vi "Append Usage.vi"(9 "Class":string, 10 "VIs":refnum<vi>[](array[refnum]), 11 "Class Relations Map":T1(c390)) -> (3 "Class Relations Map Out":T1(c390))   [LabVIEW 2019]
uses:
  <vilib>/Utility/traverseref.llb/TRef TravTarget.ctl
  <vilib>/Utility/miscctls.llb/LVMapReplaceAction.ctl
  <vilib>/Utility/traverseref.llb/VI Scripting - Traverse.lvlib
  <vilib>/Utility/Data Type/NI_Data Type.lvlib
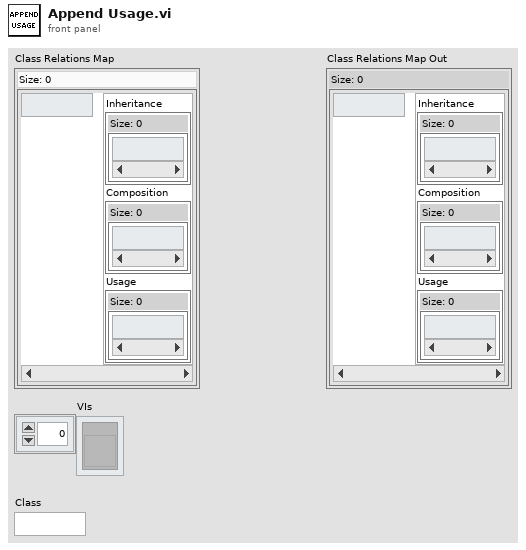
[diagram p1: front panel]
types:
  T1 = map{string, cluster{"Inheritance":set{string}, "Composition":set{string}, "Usage":set{string}}}
  T2 = typedef "TRef TravTarget.ctl" = enum16{"FP", "BD", "Other"}
  T3 = typedef "LVMapReplaceAction.ctl" = enum32{"Modify Entry only if found", "Add or Modify Entry", "Delete Entry"}
  T4 = cluster{"Inheritance":set{string}, "Composition":set{string}, "Usage":set{string}}
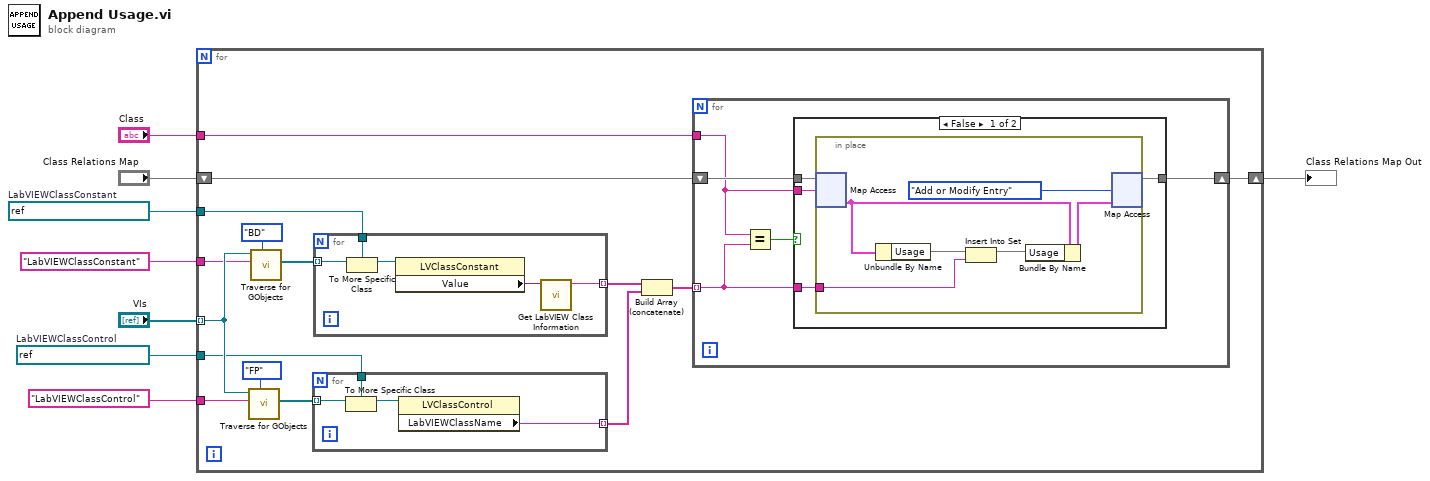
[diagram p0: block diagram]
diagram:
  w2 = refnum<vi> refnum  # LabVIEWClassControl
  w4 = refnum<vi> refnum  # LabVIEWClassConstant
  n1 = for {
    tunnel: "VIs" -> [w22] mode=indexing
    shift-right: [w14] -> w6
    shift-left: "Class Relations Map" -> [w17]
    tunnel: "Class" -> [w16]
    tunnel: w4 -> [w12]
    tunnel: "LabVIEWClassConstant" ("Class Name") -> [w11]
    tunnel: w2 -> [w10]
    tunnel: "LabVIEWClassControl" ("Class Name") -> [w9]
    n2 = call <vilib>:"Traverse for GObjects.vi"("Traverse Target"=TRef_TravTarget."FP", "Class Name"=w9, "VI Refnum"=w22) -> ("References"=w20:refnum<vi>[])  [unwired: 5 in, 3 out]
    n3 = call <vilib>:"Traverse for GObjects.vi"("Traverse Target"=TRef_TravTarget."BD", "Class Name"=w11, "VI Refnum"=w22) -> ("References"=w21:refnum<vi>[])  [unwired: 5 in, 3 out]
    n4 = for {
      tunnel: w20 -> [w42] mode=indexing
      tunnel: [w41] -> w19 mode=indexing
      tunnel: w10 -> [w40]
      n5 = To More Specific Class(target class=w40, reference=w42) -> (specific class reference=w43:refnum<vi>)  [unwired: 1 in, 1 out]
      n6 = property class="LVClassControl"(reference=w43) -> ("LabVIEWClassName"=w41:string)  [unwired: 1 in, 2 out]
    }
    n7 = for {
      tunnel: w21 -> [w47] mode=indexing
      tunnel: [w45] -> w13 mode=indexing
      tunnel: w12 -> [w44]
      n8 = To More Specific Class(target class=w44, reference=w47) -> (specific class reference=w48:refnum<vi>)  [unwired: 1 in, 1 out]
      n9 = property class="LVClassConstant"(reference=w48) -> ("Value"=w46:variant)  [unwired: 1 in, 2 out]
      n10 = call <vilib>:"Get LabVIEW Class Information.vi"("variant"=w46) -> ("LabVIEW class file name"=w45:string)  [unwired: 8 in, 2 out]
    }
    n11 = Build Array (concatenate)(w13, w19) -> (w15:string[])
    n12 = for {
      tunnel: w16 -> [w26]
      tunnel: w15 -> [w25] mode=indexing
      shift-right: [w27] -> w14
      shift-left: w17 -> [w28]
      n13 = Equal?(x=w26, y=w25) -> (x = y?=w24:bool)
      n14 = case shown="False" w24 {
        tunnel: w28 -> [w32 w39]
        tunnel: [w31 w39] -> w27
        tunnel: w26 -> [w30 _]
        tunnel: w25 -> [w29 _]
        frame False {
          n15 = in-place {
            in-place-border: w29 -> [w33]
            n16 = in-place-map #1(w32, w30) -> (w36:T4)  [unwired: 1 in, 1 out]
            n17 = Unbundle By Name(w36) -> ("Usage"=w35:set{string})
            n18 = Insert Into Set(10:w33, 11:w35) -> (3:w37:set{string})  [unwired: 1 out]
            n19 = Bundle By Name(cluster=w36, "Usage"=w37) -> (w34:T4)
            n20 = in-place-map #1(w34, LVMapReplaceAction."Add or Modify Entry" ("action")) -> (w31:T1)  [unwired: 2 out]
          }
        }
        frame True {
        }
      }
    }
  }
  "Class Relations Map Out" <- w6
